vi "Test Plan - Save Log (SubVI).vi"(7 "Data":T2 {"Others"."SC"."Load" format="%#_13g"; "Others"."SC"."Load.Time Stamp" format="%<%H:%M:%S>T"; "Others"."IC"."load" format="%#_13g"; "Custom"."Time Stamp" format="%<%H:%M:%S>T"}, 8 "error in (no error)":errorcluster, 9 "Load?":bool, 10 "Test Type":T1 items=["Please Select", "Triaxial Shear", "Triaxial UU", "Shearbox", "Permeability", "Consolidation (Stepped Loading)/Swelling/UCT", "Saturation (Incremental)/ Isotropic Consolidation", "User Defined"], 11 "path in":path) -> (0 "error out":errorcluster, 1 "Tab":u16[](array[numeric]), 2 "Test Type out":u16, 3 "path out":path, 4 "Condition":u16, 5 "Data Out":T2 {"Others"."SC"."Load" format="%#_13g"; "Others"."SC"."Load.Time Stamp" format="%<%H:%M:%S>T"; "Others"."IC"."load" format="%#_13g"; "Custom"."Time Stamp" format="%<%H:%M:%S>T"})   [LabVIEW 2019]
uses:
  Controls/SaveLog - Data.ctl
  Controls/Station - Test Type.ctl
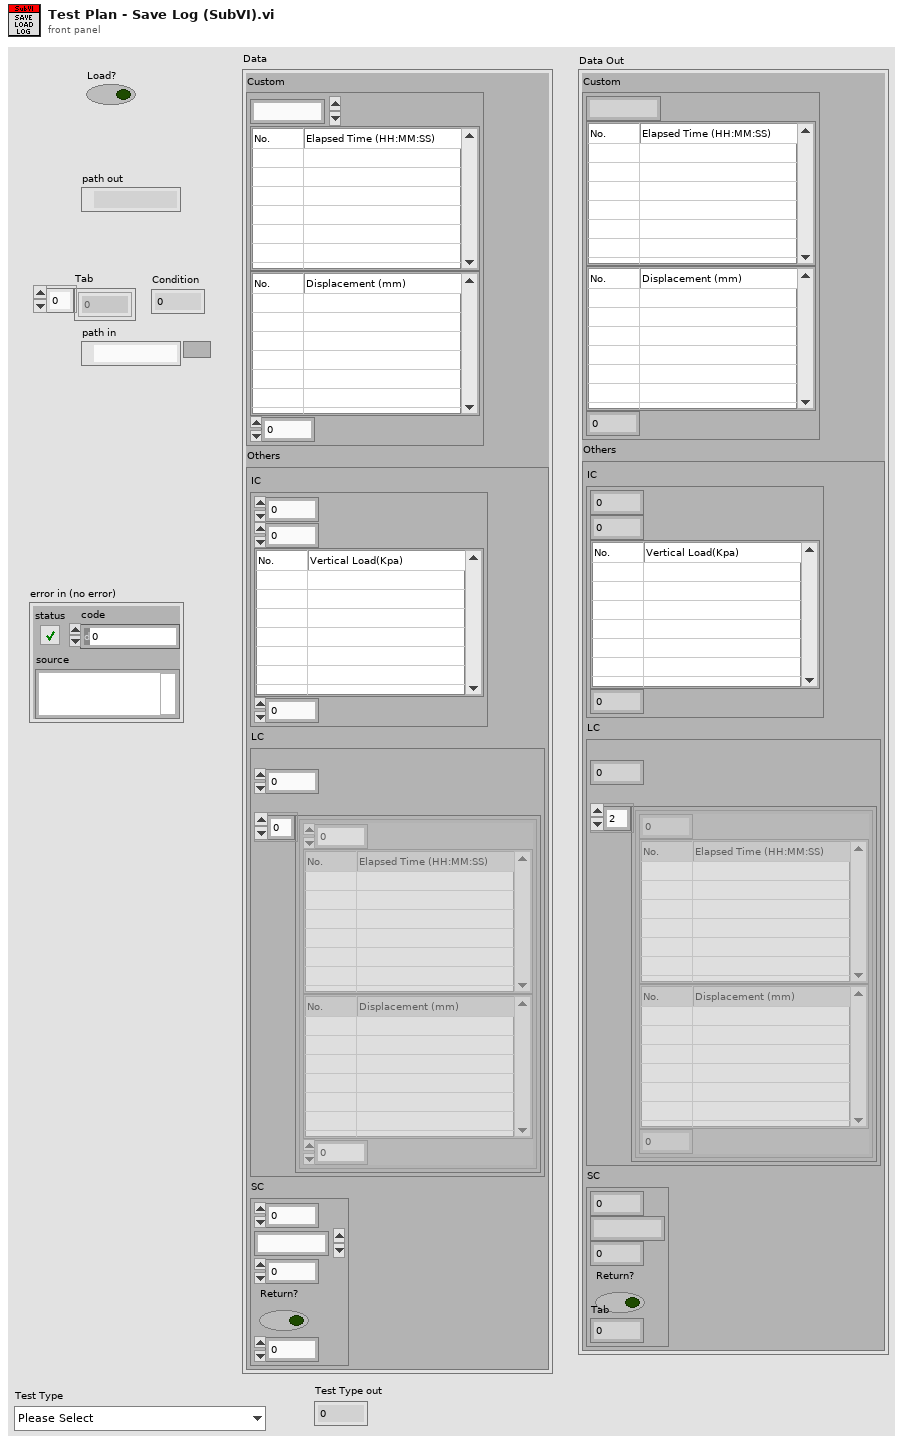
[diagram p1: front panel]
types:
  T1 = typedef "Station - Test Type.ctl" = u16
  T2 = typedef "SaveLog - Data.ctl" = cluster{"Custom":cluster{"Time Stamp":timestamp, "CustomTime":string[][], "CustomDisp":string[][], "Tab":u16}, "Others":cluster{"IC":cluster{"Numeric":u32, "load":dbl, "Custom Load":string[][], "Tab":u16}, "LC":cluster{"Set":u16, "Log data":cluster{"Numeric":u32, "CustomTime":string[][], "CustomDisp":string[][], "Tab":u16}[]}, "SC":cluster{"Max.Time Stamp":u32, "Load.Time Stamp":timestamp, "Load":dbl, "Return?":bool, "Tab":u16}}}
  T3 = enum16{"open", "replace", "create", "open or create", "replace or create", "replace or create with confirmation"}
  T4 = cluster{"Time Stamp":timestamp, "CustomTime":string[][], "CustomDisp":string[][], "Tab":u16}
  T5 = cluster{"Numeric":u32, "load":dbl, "Custom Load":string[][], "Tab":u16}
  T6 = cluster{"Set":u16, "Log data":cluster{"Numeric":u32, "CustomTime":string[][], "CustomDisp":string[][], "Tab":u16}[]}
  T7 = cluster{"Max.Time Stamp":u32, "Load.Time Stamp":timestamp, "Load":dbl, "Return?":bool, "Tab":u16}
  T8 = cluster{"Numeric":u32, "CustomTime":string[][], "CustomDisp":string[][], "Tab":u16}[]
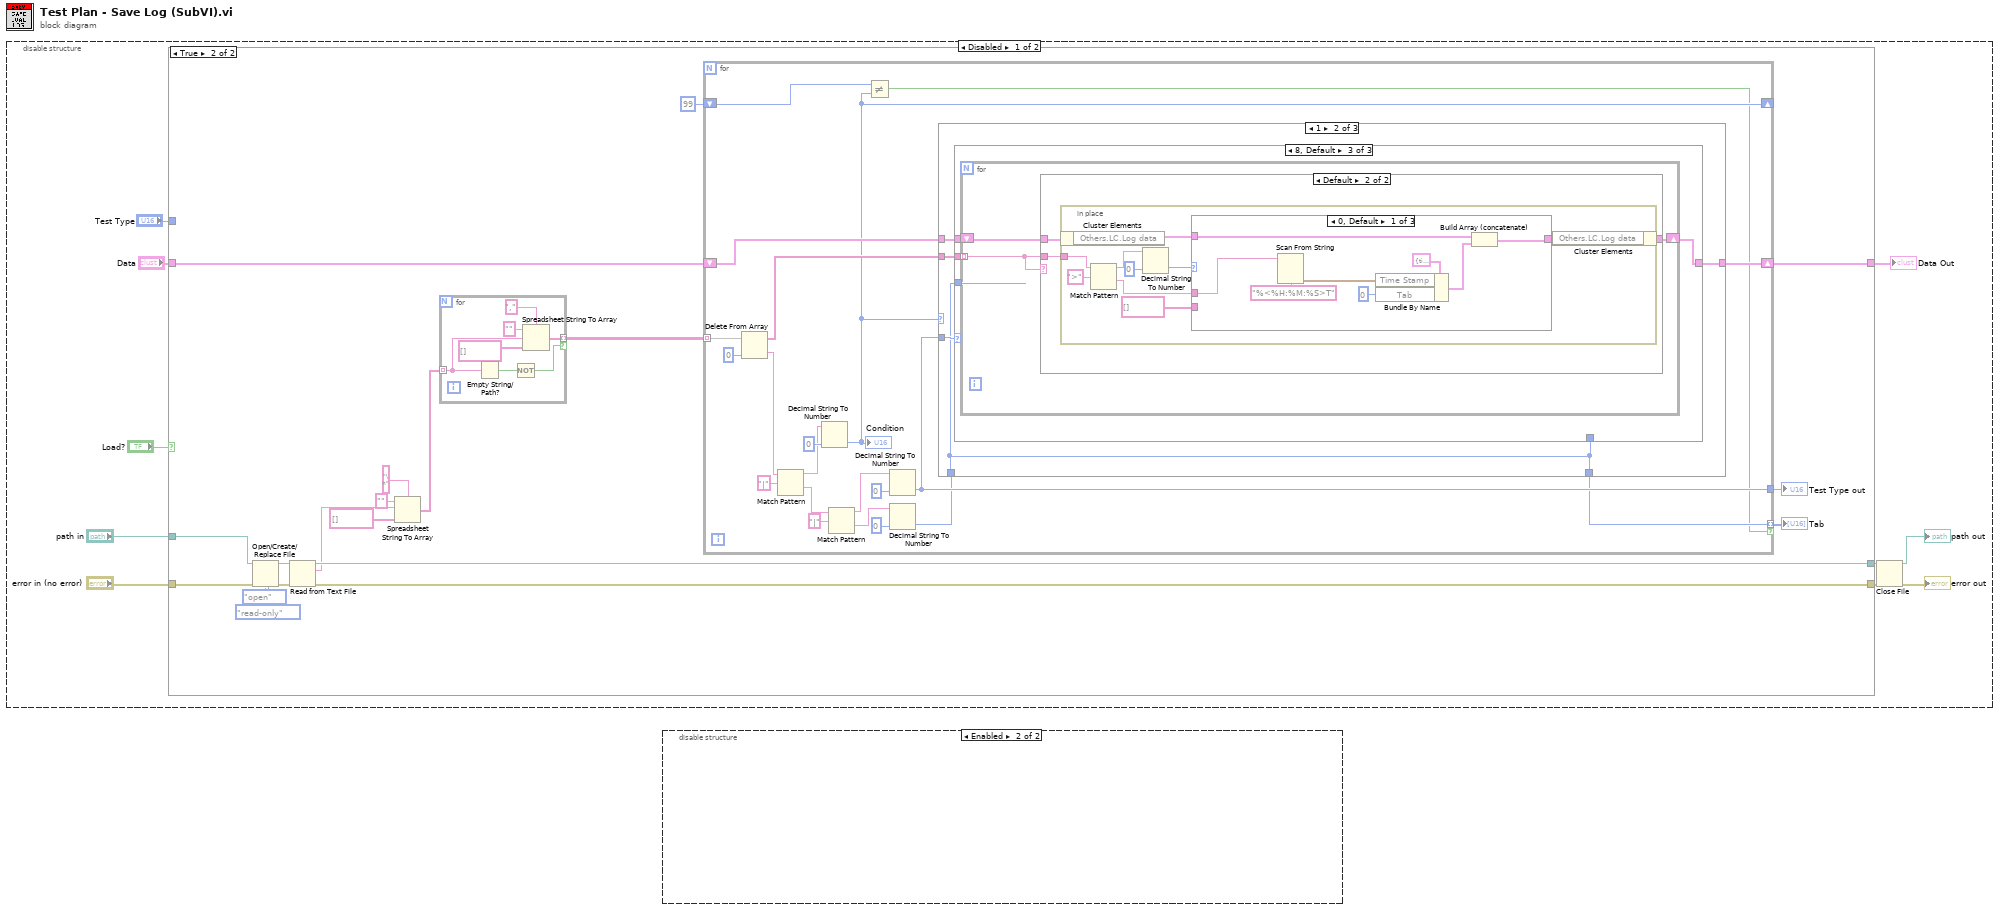
[diagram p0: block diagram]
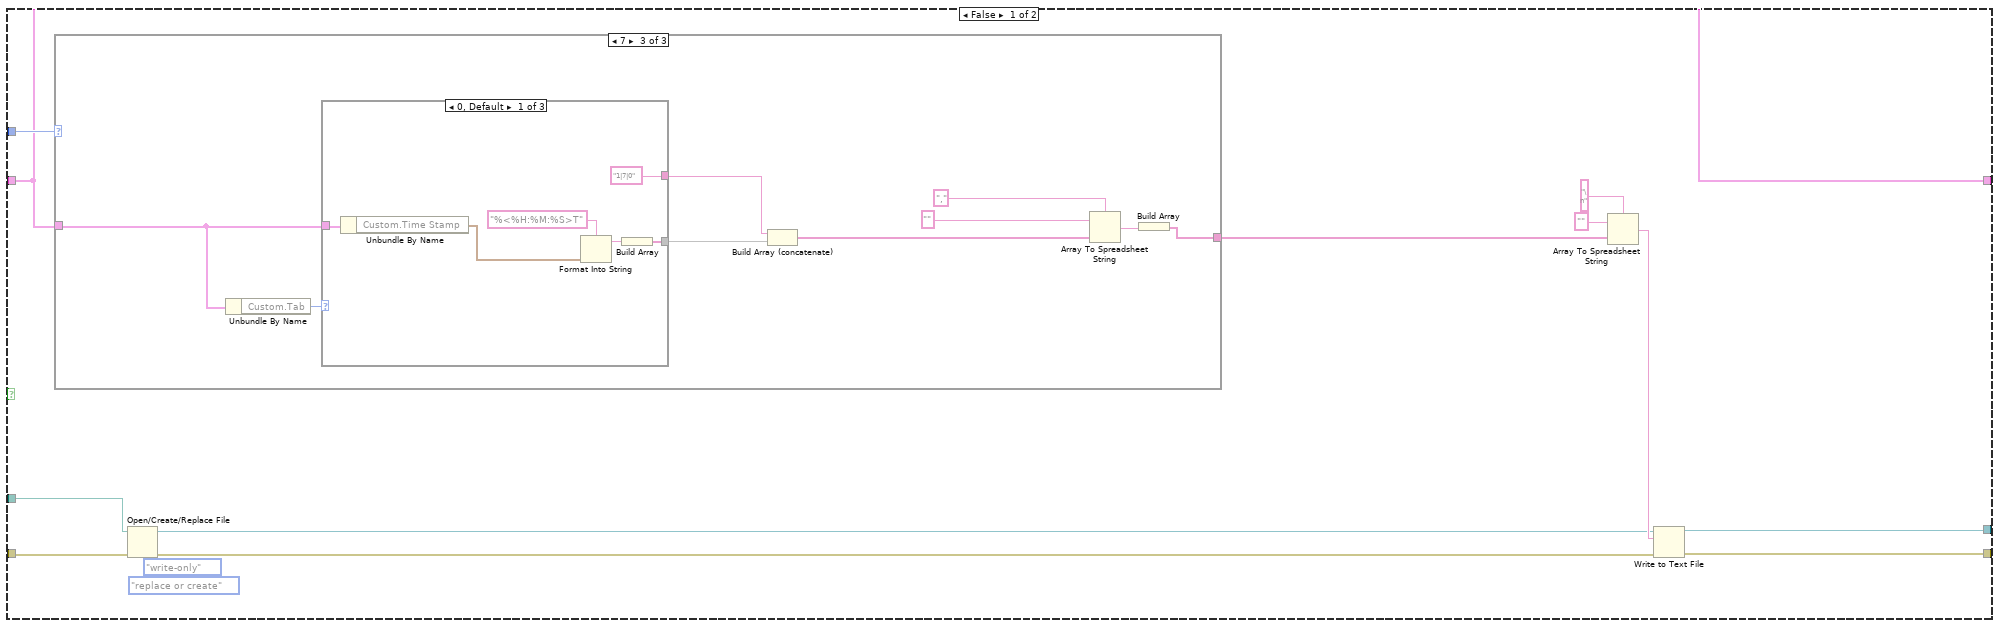
[diagram p2: hidden frame]
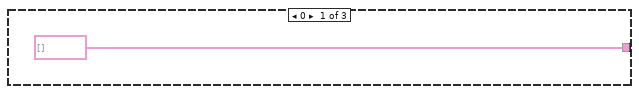
[diagram p3: hidden frame]
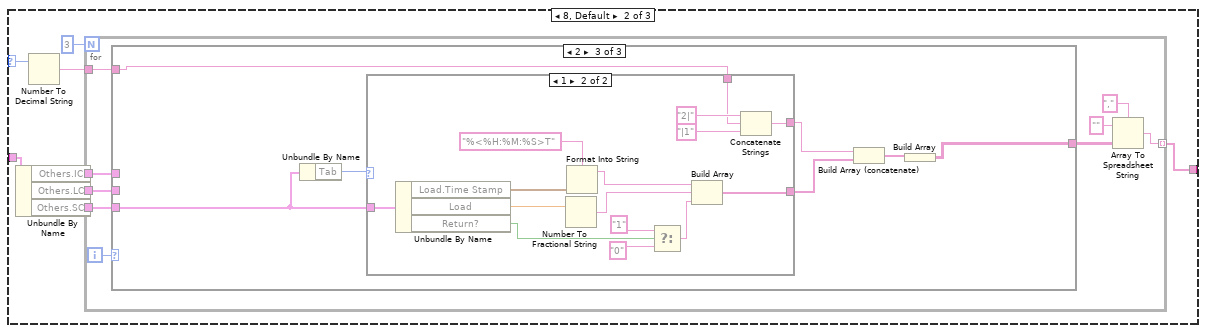
[diagram p4: hidden frame]
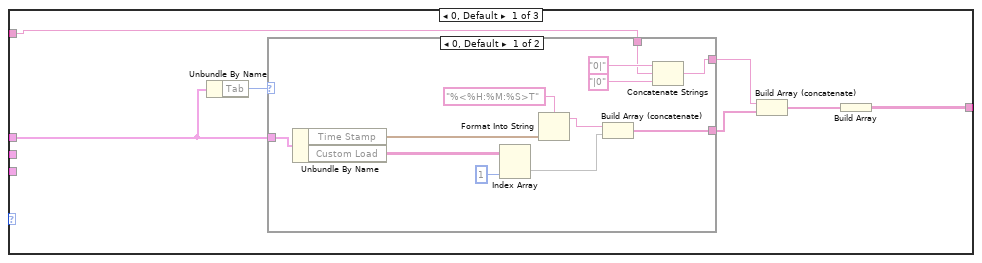
[diagram p5: hidden frame]
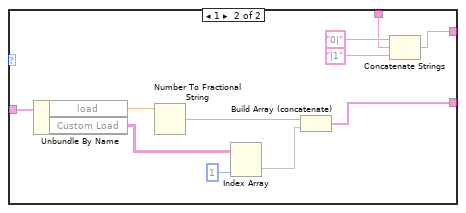
[diagram p6: hidden frame]
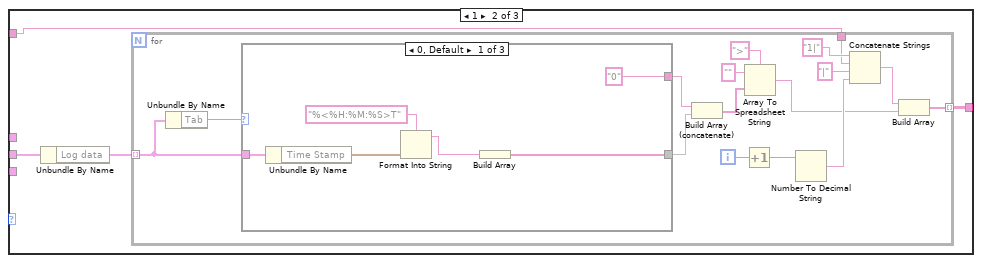
[diagram p7: hidden frame]
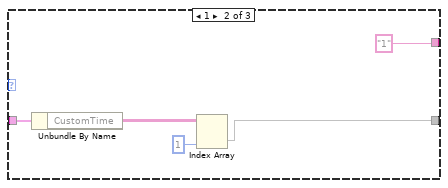
[diagram p8: hidden frame]
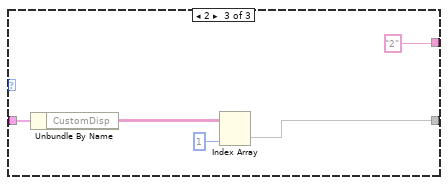
[diagram p9: hidden frame]
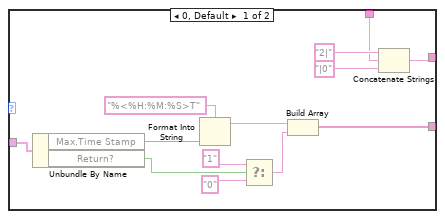
[diagram p10: hidden frame]
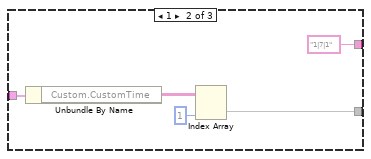
[diagram p11: hidden frame]
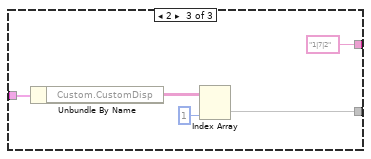
[diagram p12: hidden frame]
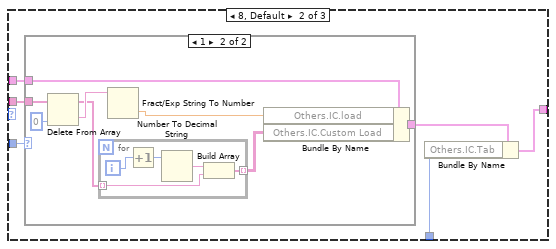
[diagram p14: hidden frame]
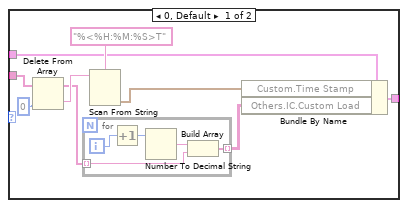
[diagram p15: hidden frame]
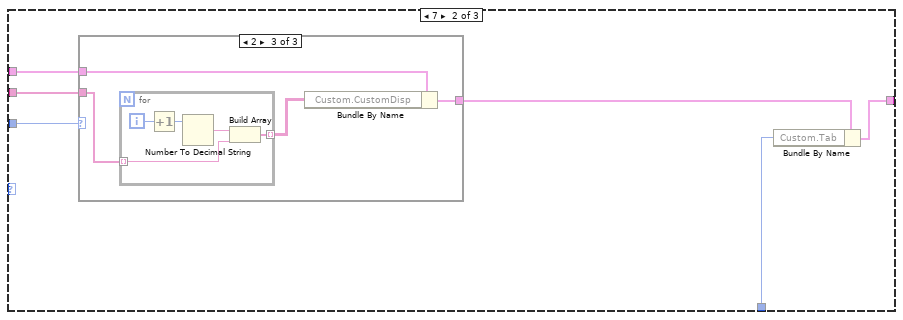
[diagram p18: hidden frame]
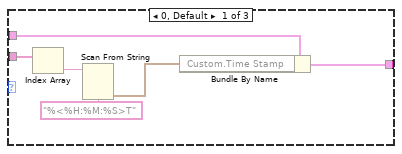
[diagram p19: hidden frame]
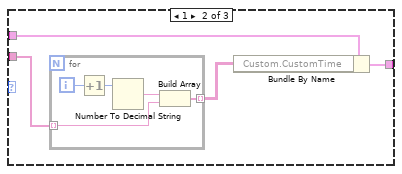
[diagram p20: hidden frame]
diagram:
  n1 = disable-structure shown="Disabled" {
    frame Disabled {
      n2 = case shown="True" "Load?" {
        tunnel: [w24 w187] -> w9
        tunnel: [w23 w186] -> w7
        tunnel: "Test Type" -> [w18 _]
        tunnel: "Data" -> [w17 w181]
        tunnel: [w17 w180] -> w4
        tunnel: "error in (no error)" -> [w13 w179]
        tunnel: "path in" -> [w14 w176]
        frame False {
          n3 = case shown="7" w18 {
            selector: w18 -> [_ w27 _]
            tunnel: w17 -> [_ w33 w151]
            tunnel: [string[] [] ("CustomDisp") w28 w144] -> w22
            frame 0 {
            }
            frame 8, Default {
              n4 = Unbundle By Name(w33) -> ("Others.IC"=w32:T5, "Others.LC"=w30:T6, "Others.SC"=w29:T7)
              n5 = Number To Decimal String(number=w27) -> (decimal integer string=w26:string)  [unwired: 1 in]
              n6 = for {
                N: 3 -> [_]
                tunnel: w32 -> [w42]
                tunnel: w30 -> [w40]
                tunnel: w29 -> [w39]
                tunnel: [w36] -> w28 mode=indexing
                tunnel: w26 -> [w34]
                i -> [w41]
                n7 = case shown="2" w41 {
                  tunnel: w42 -> [w49 _ _]
                  tunnel: w40 -> [_ w75 _]
                  tunnel: w39 -> [_ _ w114]
                  tunnel: [w44 w74 w110] -> w35
                  tunnel: w34 -> [w43 w73 w109]
                  frame 0, Default {
                    n8 = Unbundle By Name(w49) -> ("Tab"=w48:u16)
                    n9 = case shown="0, Default" w48 {
                      tunnel: w49 -> [w61 w72]
                      tunnel: [w50 w62] -> w47
                      tunnel: [w57 w69] -> w46
                      tunnel: w43 -> [w51 w63]
                      frame 0, Default {
                        n10 = Unbundle By Name(w61) -> ("Time Stamp"=w59:timestamp, "Custom Load"=w55:string[][])
                        n11 = Index Array(array=w55, index (col)=1 ("disabled index (col)")) -> (element=w54:string[])  [unwired: 1 in]
                        n12 = Format Into String(format string="%<%H:%M:%S>T", w59) -> (resulting string=w58:string)  [unwired: 2 in, 1 out]
                        n13 = Build Array (concatenate)(w58, w54) -> (w57:string[])
                        n14 = Concatenate Strings("0|", w51, "|0") -> (w50:string)
                      }
                      frame 1 {
                        n15 = Unbundle By Name(w72) -> ("load"=w71:dbl, "Custom Load"=w67:string[][])
                        n16 = Number To Fractional String(number=w71) -> (F-format string=w70:string)  [unwired: 3 in]
                        n17 = Index Array(array=w67, index (col)=1 ("disabled index (col)")) -> (element=w66:string[])  [unwired: 1 in]
                        n18 = Build Array (concatenate)(w70, w66) -> (w69:string[])
                        n19 = Concatenate Strings("0|", w63, "|1") -> (w62:string)
                      }
                    }
                    n20 = Build Array (concatenate)(w47, w46) -> (w45:string[])
                    n21 = Build Array(w45) -> (w44:string[][])
                  }
                  frame 1 {
                    n22 = Unbundle By Name(w75) -> ("Log data"=w76:T8)
                    n23 = for {
                      tunnel: w76 -> [w92] mode=indexing
                      tunnel: [w80] -> w74 mode=indexing
                      tunnel: w73 -> [w78]
                      i -> [w88]
                      n24 = Unbundle By Name(w92) -> ("Tab"=w91:u16)
                      n25 = case shown="0, Default" w91 {
                        tunnel: w92 -> [w98 w103 w108]
                        tunnel: ["0" "1" "2"] -> w90
                        tunnel: [w93 w100 w105] -> w89
                        frame 0, Default {
                          n26 = Unbundle By Name(w98) -> ("Time Stamp"=w96:timestamp)
                          n27 = Format Into String(format string="%<%H:%M:%S>T", w96) -> (resulting string=w95:string)  [unwired: 2 in, 1 out]
                          n28 = Build Array(w95) -> (w93:string[])
                        }
                        frame 1 {
                          n29 = Unbundle By Name(w103) -> ("CustomTime"=w101:string[][])
                          n30 = Index Array(array=w101, index (col)=1 ("disabled index (col)")) -> (element=w100:string[])  [unwired: 1 in]
                        }
                        frame 2 {
                          n31 = Unbundle By Name(w108) -> ("CustomDisp"=w106:string[][])
                          n32 = Index Array(array=w106, index (col)=1 ("disabled index (col)")) -> (element=w105:string[])  [unwired: 1 in]
                        }
                      }
                      n33 = Build Array (concatenate)(w90, w89) -> (w85:string[])
                      n34 = Increment(x=w88) -> (x+1=w82:i32)
                      n35 = Array To Spreadsheet String(delimiter (Tab)=">", array=w85, 3:"" ("format string")) -> (spreadsheet string=w81:string)
                      n36 = Number To Decimal String(number=w82) -> (decimal integer string=w84:string)  [unwired: 1 in]
                      n37 = Concatenate Strings("1|", w78, "|" ("string"), w84) -> (w83:string)
                      n38 = Build Array(w83, w81) -> (w80:string[])
                    }
                  }
                  frame 2 {
                    n39 = Unbundle By Name(w114) -> ("Tab"=w115:u16)
                    n40 = case shown="1" w115 {
                      tunnel: w114 -> [w128 w143]
                      tunnel: [w124 w133] -> w112
                      tunnel: [w116 w130] -> w113
                      tunnel: w109 -> [w117 w129]
                      frame 0, Default {
                        n41 = Unbundle By Name(w128) -> ("Max.Time Stamp"=w126:u32, "Return?"=w123:bool)
                        n42 = Format Into String(format string="%<%H:%M:%S>T", w126) -> (resulting string=w125:string)  [unwired: 2 in, 1 out]
                        n43 = Select(t="1", s=w123, f="0") -> (s? t:f=w122:string)
                        n44 = Build Array(w125, w122) -> (w124:string[])
                        n45 = Concatenate Strings("2|", w117, "|0") -> (w116:string)
                      }
                      frame 1 {
                        n46 = Unbundle By Name(w143) -> ("Load.Time Stamp"=w141:timestamp, "Load"=w139:dbl, "Return?"=w135:bool)
                        n47 = Number To Fractional String(number=w139) -> (F-format string=w138:string)  [unwired: 3 in]
                        n48 = Format Into String(format string="%<%H:%M:%S>T", w141) -> (resulting string=w140:string)  [unwired: 2 in, 1 out]
                        n49 = Select(t="1", s=w135, f="0") -> (s? t:f=w134:string)
                        n50 = Build Array(w140, w138, w134) -> (w133:string[])
                        n51 = Concatenate Strings("2|", w129, "|1") -> (w130:string)
                      }
                    }
                    n52 = Build Array (concatenate)(w113, w112) -> (w111:string[])
                    n53 = Build Array(w111) -> (w110:string[][])
                  }
                }
                n54 = Array To Spreadsheet String(delimiter (Tab)=",", array=w35, 3:"" ("format string")) -> (spreadsheet string=w36:string)
              }
            }
            frame 7 {
              n55 = Unbundle By Name(w151) -> ("Custom.Tab"=w152:u16)
              n56 = case shown="0, Default" w152 {
                tunnel: [w156 w162 w167] -> w150
                tunnel: w151 -> [w155 w161 w166]
                tunnel: ["1|7|0" ("format string") "1|7|1" ("format string") "1|7|2" ("format string")] -> w149
                frame 0, Default {
                  n57 = Unbundle By Name(w155) -> ("Custom.Time Stamp"=w154:timestamp)
                  n58 = Format Into String(format string="%<%H:%M:%S>T", w154) -> (resulting string=w157:string)  [unwired: 2 in, 1 out]
                  n59 = Build Array(w157) -> (w156:string[])
                }
                frame 1 {
                  n60 = Unbundle By Name(w161) -> ("Custom.CustomTime"=w160:string[][])
                  n61 = Index Array(array=w160, index (col)=1 ("disabled index (col)")) -> (element=w162:string[])  [unwired: 1 in]
                }
                frame 2 {
                  n62 = Unbundle By Name(w166) -> ("Custom.CustomDisp"=w165:string[][])
                  n63 = Index Array(array=w165, index (col)=1 ("disabled index (col)")) -> (element=w167:string[])  [unwired: 1 in]
                }
              }
              n64 = Build Array (concatenate)(w149, w150) -> (w145:string[])
              n65 = Array To Spreadsheet String(delimiter (Tab)=",", array=w145, 3:"" ("format string")) -> (spreadsheet string=w146:string)
              n66 = Build Array(w146) -> (w144:string[])
            }
          }
          n67 = Open/Create/Replace File(file path (use dialog)=w14, error in=w13, operation (0:open)=T3."replace or create", access (0:read/write)=enum16{"read/write", "read-only", "write-only"}."write-only") -> (refnum out=w11:refnum<file>, error out=w12:errorcluster)  [unwired: 2 in, 1 out]
          n68 = Array To Spreadsheet String(delimiter (Tab)="\n", array=w22, 3:"" ("format string")) -> (spreadsheet string=w21:string)
          n69 = Write to Text File(file (use dialog)=w11, text=w21, error in=w12) -> (refnum out=w24:refnum<file>, error out=w23:errorcluster)  [unwired: 1 in, 1 out]
        }
        frame True {
          n70 = Open/Create/Replace File(file path (use dialog)=w176, error in=w179, operation (0:open)=T3."open", access (0:read/write)=enum16{"read/write", "read-only", "write-only"}."read-only") -> (refnum out=w174:refnum<file>, error out=w175:errorcluster)  [unwired: 2 in, 1 out]
          n71 = Read from Text File(file (use dialog)=w174, error in=w175) -> (refnum out=w187:refnum<file>, text=w185:string, error out=w186:errorcluster)  [unwired: 2 in, 1 out]
          n72 = Spreadsheet String To Array(delimiter (Tab)="\n", format string="", spreadsheet string=w185, array type (2D Dbl)=string[] []) -> (array=w173:string[])
          n73 = for {
            tunnel: w173 -> [w385] mode=indexing
            tunnel: [w384] -> w172 mode=indexing if=w389
            n74 = Empty String/Path?(string/path=w385) -> (empty?=w390:bool)
            n75 = Not(x=w390) -> (.not. x?=w389:bool)
            n76 = Spreadsheet String To Array(delimiter (Tab)=",", format string="", spreadsheet string=w385, array type (2D Dbl)=string[] []) -> (array=w384:string[])
          }
          n77 = for {
            shift-right: [w201] -> w180
            shift-left: w181 -> [w203]
            tunnel: w172 -> [w194] mode=indexing
            tunnel: [w193] -> w169
            tunnel: [w191] -> w171 mode=indexing if=w188
            shift-right: [w190] -> _
            shift-left: u16 99 -> [w189]
            n78 = Delete From Array(array=w194, index=0) -> (deleted portion=w207:string, array with subset deleted=w202:string[])  [unwired: 1 in]
            n79 = Match Pattern(string=w207, regular expression="|") -> (before substring=w195:string, after substring=w199:string)  [unwired: 1 in, 2 out]
            n80 = Decimal String To Number(string=w195, default (0L)=u16 0 ("default (0 I32)")) -> (number=w190:u16)  [unwired: 1 in, 1 out]
            "Condition" <- w190
            n81 = Match Pattern(string=w199, regular expression="|") -> (before substring=w198:string, after substring=w197:string)  [unwired: 1 in, 2 out]
            n82 = Not Equal?(x=w189, y=w190) -> (x != y?=w188:bool)
            n83 = Decimal String To Number(string=w198, default (0L)=u16 0 ("default (0 I32)")) -> (number=w193:u16)  [unwired: 1 in, 1 out]
            n84 = Decimal String To Number(string=w197, default (0L)=u16 0 ("default (0 I32)")) -> (number=w192:u16)  [unwired: 1 in, 1 out]
            n85 = case shown="1" w190 {
              tunnel: w193 -> [w213 w253 w348]
              tunnel: w203 -> [w211 w252 w346]
              tunnel: w202 -> [w212 w251 w347]
              tunnel: [w210 w250 w345] -> w201
              tunnel: w192 -> [w209 w249 w344]
              tunnel: [w209 w249 w344] -> w191
              frame 0, Default {
                n86 = case shown="0" w213 {
                  tunnel: w212 -> [_ w219 _]
                  tunnel: w211 -> [w214 w218 w248]
                  tunnel: [w214 w216 w248] -> w210
                  tunnel: w209 -> [_ w220 _]
                  tunnel: w209 -> [_ w215 _]
                  frame 0 {
                  }
                  frame 8, Default {
                    n87 = case shown="1" w220 {
                      tunnel: w219 -> [w224 w238]
                      tunnel: w218 -> [w228 w241]
                      tunnel: [w226 w242] -> w217
                      frame 0, Default {
                        n88 = Delete From Array(array=w224, index=0) -> (deleted portion=w222:string, array with subset deleted=w221:string[])  [unwired: 1 in]
                        n89 = for {
                          tunnel: w221 -> [w232] mode=indexing
                          tunnel: [w231] -> w225 mode=indexing
                          i -> [w234]
                          n90 = Increment(x=w234) -> (x+1=w230:i32)
                          n91 = Number To Decimal String(number=w230) -> (decimal integer string=w233:string)  [unwired: 1 in]
                          n92 = Build Array(w233, w232) -> (w231:string[])
                        }
                        n93 = Scan From String(format string="%<%H:%M:%S>T", input string=w222) -> (output 1=w227:timestamp)  [unwired: 3 in, 3 out]
                        n94 = Bundle By Name(cluster=w228, "Custom.Time Stamp"=w227, "Others.IC.Custom Load"=w225) -> (w226:T2)
                      }
                      frame 1 {
                        n95 = Delete From Array(array=w238, index=0) -> (deleted portion=w236:string, array with subset deleted=w235:string[])  [unwired: 1 in]
                        n96 = for {
                          tunnel: w235 -> [w245] mode=indexing
                          tunnel: [w244] -> w239 mode=indexing
                          i -> [w247]
                          n97 = Increment(x=w247) -> (x+1=w243:i32)
                          n98 = Number To Decimal String(number=w243) -> (decimal integer string=w246:string)  [unwired: 1 in]
                          n99 = Build Array(w246, w245) -> (w244:string[])
                        }
                        n100 = Fract/Exp String To Number(string=w236) -> (number=w240:dbl)  [unwired: 3 in, 1 out]
                        n101 = Bundle By Name(cluster=w241, "Others.IC.load"=w240, "Others.IC.Custom Load"=w239) -> (w242:T2)
                      }
                    }
                    n102 = Bundle By Name(cluster=w217, "Others.IC.Tab"=w215) -> (w216:T2)
                  }
                  frame 7 {
                  }
                }
              }
              frame 1 {
                n103 = case shown="8, Default" w253 {
                  tunnel: w249 -> [_ w260 _]
                  tunnel: w252 -> [w254 w259 w287]
                  tunnel: w251 -> [_ w258 w286]
                  tunnel: [w254 w255 w285] -> w250
                  tunnel: w249 -> [_ w257 _]
                  frame 0 {
                  }
                  frame 7 {
                    n104 = case shown="2" w260 {
                      tunnel: w259 -> [w266 w270 w279]
                      tunnel: w258 -> [w265 w268 w277]
                      tunnel: [w261 w269 w278] -> w256
                      frame 0, Default {
                        n105 = Index Array(array=w265) -> (element=w263:string)  [unwired: 1 in]
                        n106 = Scan From String(format string="%<%H:%M:%S>T", input string=w263) -> (output 1=w262:timestamp)  [unwired: 3 in, 3 out]
                        n107 = Bundle By Name(cluster=w266, "Custom.Time Stamp"=w262) -> (w261:T2)
                      }
                      frame 1 {
                        n108 = for {
                          tunnel: w268 -> [w273] mode=indexing
                          tunnel: [w272] -> w267 mode=indexing
                          i -> [w275]
                          n109 = Increment(x=w275) -> (x+1=w271:i32)
                          n110 = Number To Decimal String(number=w271) -> (decimal integer string=w274:string)  [unwired: 1 in]
                          n111 = Build Array(w274, w273) -> (w272:string[])
                        }
                        n112 = Bundle By Name(cluster=w270, "Custom.CustomTime"=w267) -> (w269:T2)
                      }
                      frame 2 {
                        n113 = for {
                          tunnel: w277 -> [w282] mode=indexing
                          tunnel: [w281] -> w276 mode=indexing
                          i -> [w284]
                          n114 = Increment(x=w284) -> (x+1=w280:i32)
                          n115 = Number To Decimal String(number=w280) -> (decimal integer string=w283:string)  [unwired: 1 in]
                          n116 = Build Array(w283, w282) -> (w281:string[])
                        }
                        n117 = Bundle By Name(cluster=w279, "Custom.CustomDisp"=w276) -> (w278:T2)
                      }
                    }
                    n118 = Bundle By Name(cluster=w256, "Custom.Tab"=w257) -> (w255:T2)
                  }
                  frame 8, Default {
                    n119 = for {
                      tunnel: w286 -> [w288] mode=indexing
                      shift-right: [w289] -> w285
                      shift-left: w287 -> [w290]
                      n120 = case shown="Default" w288 {
                        tunnel: w288 -> [_ w294]
                        tunnel: w290 -> [w291 w293]
                        tunnel: [w291 w292] -> w289
                        frame "" {
                        }
                        frame Default {
                          n121 = in-place {
                            in-place-border: w294 -> [w302]
                            n122 = in-place-cluster #1(w293) -> ("Others.LC.Log data"=w297:T8)
                            n123 = Match Pattern(string=w302, regular expression=">") -> (before substring=w300:string, after substring=w298:string)  [unwired: 1 in, 2 out]
                            n124 = Decimal String To Number(string=w300, default (0L)=u16 0 ("default (0 I32)")) -> (number=w299:u16)  [unwired: 1 in, 1 out]
                            n125 = case shown="0, Default" w299 {
                              tunnel: w298 -> [w305 w315 w331]
                              tunnel: w297 -> [w311 w322 w338]
                              tunnel: [w310 w321 w337] -> w296
                              tunnel: string[] [] ("array type (2D Dbl)") -> [_ w313 w329]
                              frame 0, Default {
                                n126 = Scan From String(format string="%<%H:%M:%S>T", input string=w305) -> (output 1=w304:timestamp)  [unwired: 3 in, 3 out]
                                n127 = Bundle By Name(cluster=T4 {"Time Stamp"=timestamp(0 s since 1904-01-01), "CustomTime"=[], "CustomDisp"=[], "Tab"=0} ("new element/subarray"), "Time Stamp"=w304, "Tab"=u16 0) -> (w308:T4)
                                n128 = Build Array (concatenate)(w311, w308) -> (w310:T8)
                              }
                              frame 1 {
                                n129 = Spreadsheet String To Array(delimiter (Tab)=">", format string="", spreadsheet string=w315, array type (2D Dbl)=w313) -> (array=w314:string[])
                                n130 = for {
                                tunnel: w314 -> [w327] mode=indexing
                                tunnel: [w323] -> w312 mode=indexing
                                i -> [w326]
                                n131 = Increment(x=w326) -> (x+1=w325:i32)
                                n132 = Number To Decimal String(number=w325) -> (decimal integer string=w324:string)  [unwired: 1 in]
                                n133 = Build Array(w324, w327) -> (w323:string[])
                                }
                                n134 = Bundle By Name(cluster=T4 {"Time Stamp"=timestamp(0 s since 1904-01-01), "CustomTime"=[], "CustomDisp"=[], "Tab"=0} ("new element/subarray"), "CustomTime"=w312, "Tab"=u16 1) -> (w319:T4)
                                n135 = Build Array (concatenate)(w322, w319) -> (w321:T8)
                              }
                              frame 2 {
                                n136 = Spreadsheet String To Array(delimiter (Tab)=">", format string="", spreadsheet string=w331, array type (2D Dbl)=w329) -> (array=w330:string[])
                                n137 = for {
                                tunnel: w330 -> [w343] mode=indexing
                                tunnel: [w339] -> w328 mode=indexing
                                i -> [w342]
                                n138 = Increment(x=w342) -> (x+1=w341:i32)
                                n139 = Number To Decimal String(number=w341) -> (decimal integer string=w340:string)  [unwired: 1 in]
                                n140 = Build Array(w340, w343) -> (w339:string[])
                                }
                                n141 = Bundle By Name(cluster=T4 {"Time Stamp"=timestamp(0 s since 1904-01-01), "CustomTime"=[], "CustomDisp"=[], "Tab"=0} ("new element/subarray"), "CustomDisp"=w328, "Tab"=u16 2) -> (w335:T4)
                                n142 = Build Array (concatenate)(w338, w335) -> (w337:T8)
                              }
                            }
                            n143 = in-place-cluster #1("Others.LC.Log data"=w296) -> (w292:T2)
                          }
                        }
                      }
                    }
                  }
                }
              }
              frame 2 {
                n144 = case shown="7" w348 {
                  tunnel: w347 -> [_ w353 _]
                  tunnel: w346 -> [w349 w354 w383]
                  tunnel: [w349 w351 w383] -> w345
                  tunnel: w344 -> [_ w355 _]
                  tunnel: w344 -> [_ w350 _]
                  frame 0, Default {
                  }
                  frame 8 {
                    n145 = case shown="0, Default" w355 {
                      tunnel: w354 -> [w363 w378]
                      tunnel: w353 -> [w360 w370]
                      tunnel: [w362 w377] -> w352
                      frame 0, Default {
                        n146 = Index Array(array=w360, index=0) -> (element=w364:string)
                        n147 = Index Array(array=w360, index=1) -> (element=w357:string)
                        n148 = Scan From String(format string="%<%H:%M:%S>T", input string=w364) -> (output 1=w361:timestamp)  [unwired: 3 in, 3 out]
                        n149 = case shown="\"1\", Default" w357 {
                          tunnel: [TRUE FALSE] -> w356
                          frame "1", Default {
                          }
                          frame "0" {
                          }
                        }
                        n150 = Bundle By Name(cluster=w363, "Others.SC.Max.Time Stamp"=w361, "Others.SC.Return?"=w356) -> (w362:T2)
                      }
                      frame 1 {
                        n151 = Index Array(array=w370, index=0) -> (element=w379:string)
                        n152 = Index Array(array=w370, index=1) -> (element=w374:string)
                        n153 = Index Array(array=w370, index=2) -> (element=w369:string)
                        n154 = Scan From String(format string="%<%H:%M:%S>T", input string=w379) -> (output 1=w376:timestamp)  [unwired: 3 in, 3 out]
                        n155 = Fract/Exp String To Number(string=w374) -> (number=w373:dbl)  [unwired: 3 in, 1 out]
                        n156 = case shown="\"1\", Default" w369 {
                          tunnel: [TRUE FALSE] -> w368
                          frame "1", Default {
                          }
                          frame "0" {
                          }
                        }
                        n157 = Bundle By Name(cluster=w378, "Others.SC.Load.Time Stamp"=w376, "Others.SC.Load"=w373, "Others.SC.Return?"=w368) -> (w377:T2)
                      }
                    }
                    n158 = Bundle By Name(cluster=w352, "Others.SC.Tab"=w350) -> (w351:T2)
                  }
                  frame 7 {
                  }
                }
              }
            }
          }
          "Tab" <- w171
          "Test Type out" <- w169
        }
      }
      "Data Out" <- w4
      n159 = Close File(refnum=w9, error in=w7) -> (path=→"path out":path, error out=→"error out":errorcluster)
    }
    frame Enabled {
    }
  }
  n160 = disable-structure shown="Enabled" {
    frame Disabled {
      n161 = case shown="0, Default" {
        selector: _ -> [_ _ _]
        tunnel: _ -> [w391 w399 w408]
        tunnel: _ -> [w392 w397 w406]
        tunnel: [_ w398 w407] -> _
        frame 0, Default {
          n162 = in-place {
            in-place-border: w392 -> [w395]
            n163 = in-place-cluster #2(w391) -> ()  [unwired: 1 out]
            n164 = Index Array(array=w395) -> (element=w393)  [unwired: 1 in]
            n165 = Scan From String(format string="%<%H:%M:%S>T", input string=w393) -> ()  [unwired: 4 in, 3 out]
            n166 = in-place-cluster #2() -> ()  [unwired: 1 in, 1 out]
          }
        }
        frame 1 {
          n167 = for {
            tunnel: w397 -> [w402] mode=indexing
            tunnel: [w401] -> w396 mode=indexing
            i -> [w404]
            n168 = Increment(x=w404) -> (x+1=w400:i32)
            n169 = Number To Decimal String(number=w400) -> (decimal integer string=w403:string)  [unwired: 1 in]
            n170 = Build Array(w403, w402) -> (w401:string[])
          }
          n171 = Bundle By Name(cluster=w399, "CustomTime"=w396) -> (w398:cluster{})
        }
        frame 2 {
          n172 = for {
            tunnel: w406 -> [w411] mode=indexing
            tunnel: [w410] -> w405 mode=indexing
            i -> [w413]
            n173 = Increment(x=w413) -> (x+1=w409:i32)
            n174 = Number To Decimal String(number=w409) -> (decimal integer string=w412:string)  [unwired: 1 in]
            n175 = Build Array(w412, w411) -> (w410:string[])
          }
          n176 = Bundle By Name(cluster=w408, "CustomDisp"=w405) -> (w407:cluster{})
        }
      }
    }
    frame Enabled {
    }
  }
